vi "10TW_1WireSystem.vi"() -> ()   [LabVIEW 2013]
uses:
  shared programs/GUI_Template/GUI_master/tcp new data cluster.ctl
panel:
  in  "Filpper.Channel 10.Name::1":string
  in  "Filpper.Channel 9.Name::1":string
  in  "Position.Channel 10::1":T1(ring)
  in  "Position.Channel 9::1":T1(ring)
  in  "Filpper.Channel 8.Name::1":string
  in  "Position.Channel 8::1":T1(ring)
  in  "Filpper.Channel 7.Name::1":string
  in  "Position.Channel 7::1":T1(ring)
  in  "Position.Channel 6::1":T1(ring)
  in  "Filpper.Channel 6.Name::1":string
  in  "Position.Channel 5::1":T1(ring)
  in  "Filpper.Channel 5.Name::1":string="Beam2 Near"
  in  "Position.Channel 4::1":T1(ring)
  in  "Filpper.Channel 4.Name::1":string="Beam1 Far"
  in  "Filpper.Channel 3.Name::1":string="Beam1 Near"
  in  "Filpper.Channel 2.Name::1":string="Beam2 Far"
  in  "Position.Channel 3::1":T1(ring)
  in  "Filpper.Channel 1.Name::1":string="XH1"
  in  "Position.Channel 2::1":T1(ring)
  out "device status::1":string="Initialized"
  in  "Position.Channel 1::1":T1(ring)
  in  "stop":bool
  in  "GUIdevice 1":string="Staging1Wire"
  in  "insert tag":bool=TRUE
  # "10TW 1Wire"
  # "10TW_1WireSystem"
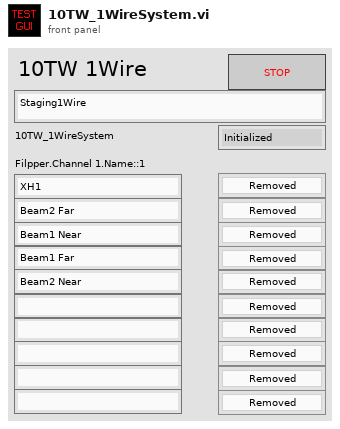
[diagram p1: front panel]
types:
  T1 = enum16{"Removed", "Inserted", "Unknown", "Moving"}
  T2 = typedef "tcp new data cluster.ctl" = cluster{"EventEnum":enum16{"new data", "connection status update"}, "Device name":string}
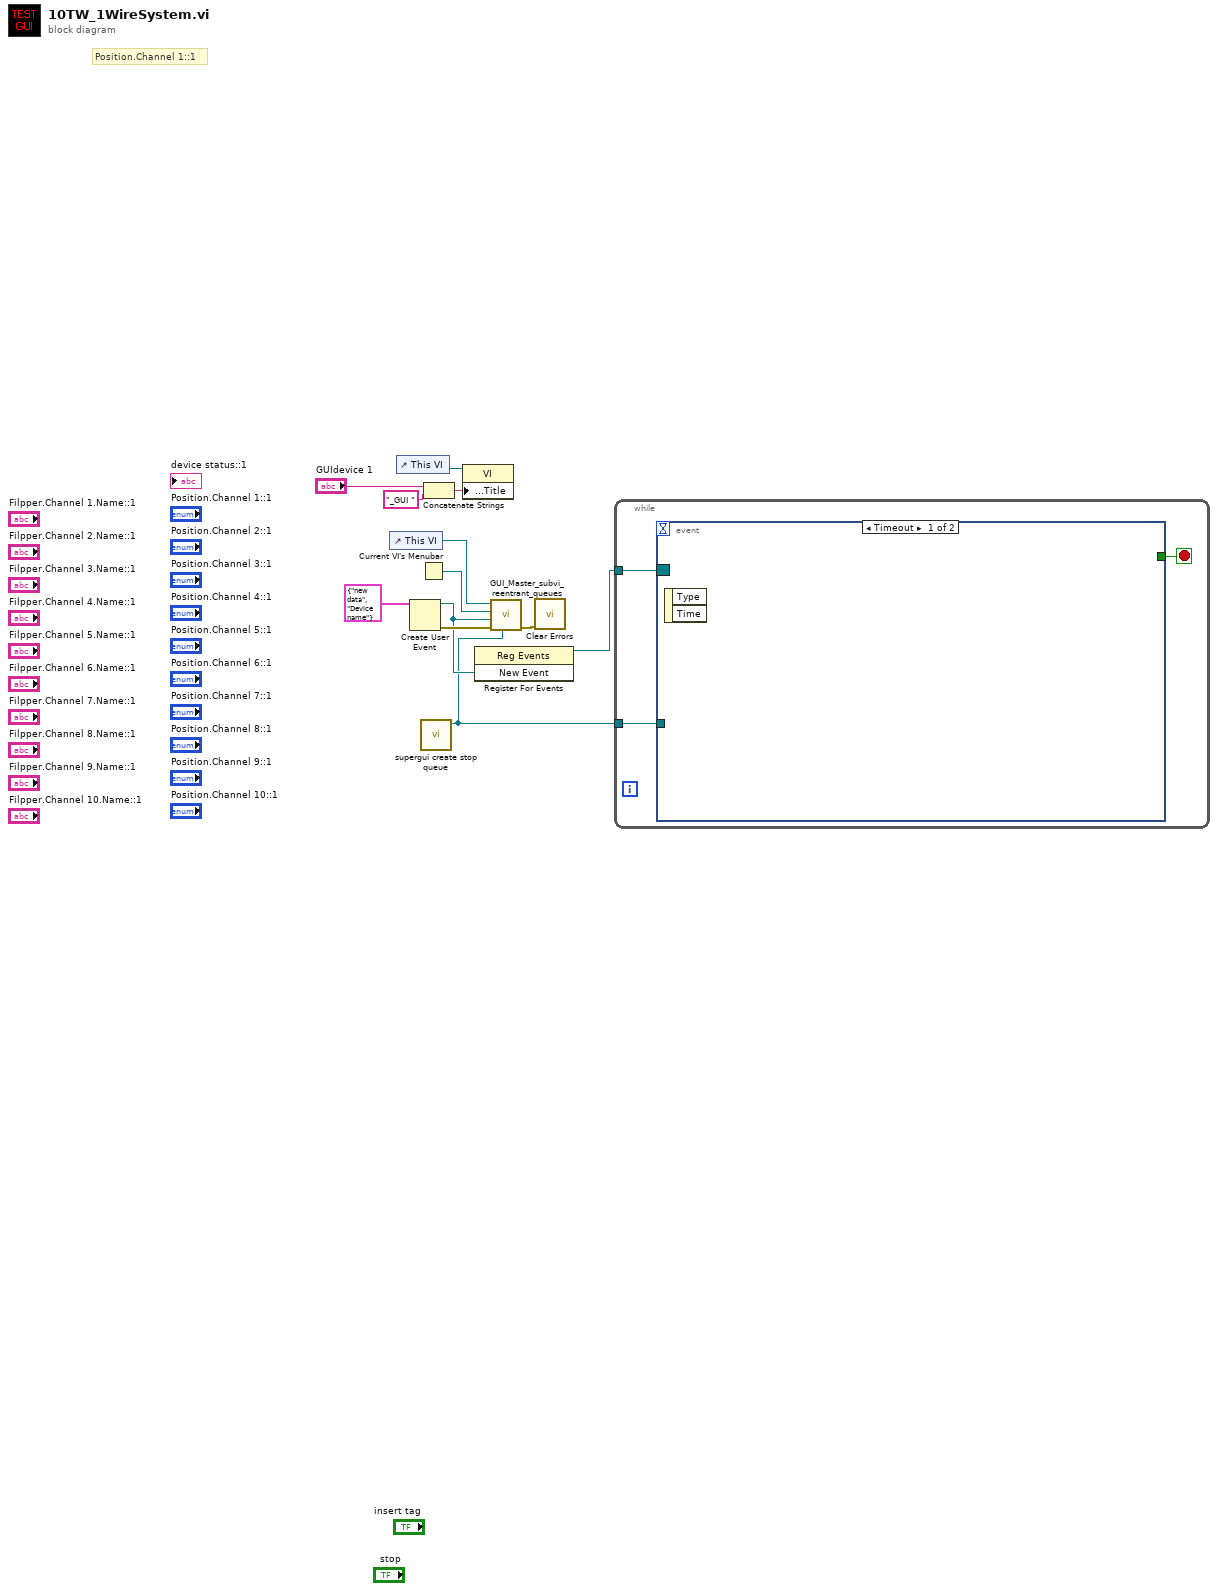
[diagram p0: block diagram]
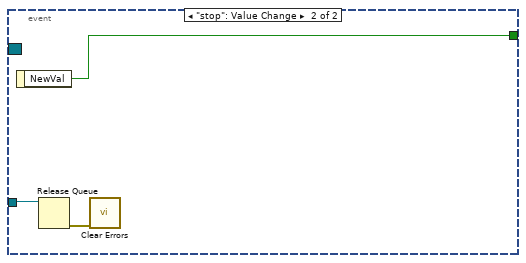
[diagram p2: hidden frame]
diagram:
  # "Position.Channel 1::1"
  n1 = control-ref of="This VI"() -> (w12:refnum<vi>)
  n2 = control-ref of="This VI"() -> (w4:refnum<vi>)
  n3 = Create User Event(user event datatype=T2 {"EventEnum"=enum."new data", "Device name"="Device name"} ("New Event")) -> (user event=w7:refnum<user-event>, error out=w9:errorcluster)  [unwired: 1 in]
  n4 = Current VI's Menubar() -> (w11:refnum<k9>)
  n5 = call "supergui create stop queue.vi"() -> ("STOP Queue out"=w5:refnum<queue>)  [unwired: 11 in]
  n6 = Concatenate Strings("GUIdevice 1", "_GUI ") -> (w3:string)
  n7 = property class="VI"(reference=w4, "Front Panel.Title"=w3) -> ()  [unwired: 1 in, 2 out]
  n8 = register-events(w7) -> (reference out=w6:refnum<event-registration>)  [unwired: 2 in, 1 out]
  n9 = call "GUI_Master_subvi_reentrant_queues.vi"("STOP Queue in"=w5, "error in (no error)"=w9, "tcp data event"=w7, "Caller menu reference"=w11, "Caller VI ref"=w12) -> ("error out"=w8:errorcluster)  [unwired: 6 in]
  n10 = call <vilib>:"Clear Errors.vi"("error in (no error)"=w8) -> ()  [unwired: 6 in, 1 out]
  n11 = while {
    tunnel: w6 -> [w15]
    tunnel: w5 -> [w13]
    stop <- w14 stop-if-true
    n12 = event shown="[0] Timeout" {
      selector: w15 -> [_ _]
      dyn-events: _ -> [_ _]
      timeout: _ -> [_ _]
      tunnel: [_ w18] -> w14
      tunnel: w13 -> [_ w17]
      event Timeout {
        n13 = event-data() -> ()  [unwired: 1 in, 2 out]
      }
      event "stop": Value Change {
        n14 = event-data() -> ("NewVal"=w18:bool)  [unwired: 1 in]
        n15 = Release Queue(queue=w17) -> (error out=w16:errorcluster)  [unwired: 2 in, 2 out]
        n16 = call <vilib>:"Clear Errors.vi"("error in (no error)"=w16) -> ()  [unwired: 6 in, 1 out]
      }
    }
  }
